vi "总圈数判定.vi"(0 "总圈数":sgl, 1 "总圈数":cluster{"下限":dbl, "上限":dbl}, 3 "错误输入":errorcluster) -> (8 "OK":bool, 10 "错误输出":errorcluster)   [LabVIEW 2018]
uses:
  Global_Variable/Global.vi
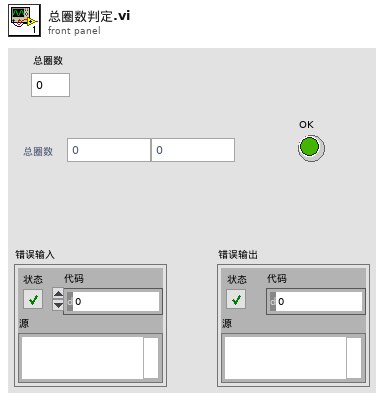
[diagram p1: front panel]
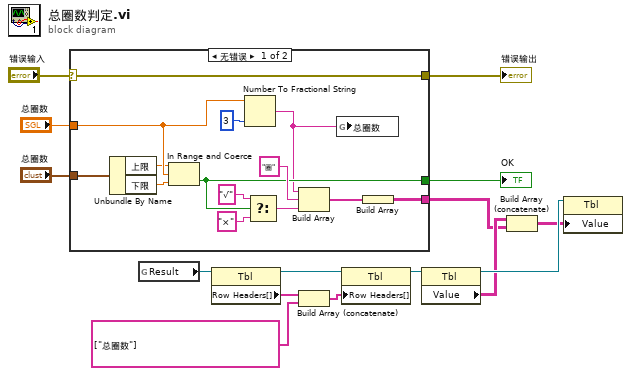
[diagram p0: block diagram]
diagram:
  n1 = case shown="无错误" "错误输入" {
    selector: "错误输入" -> [w22 w30]
    tunnel: [w22 w30] -> w14
    tunnel: [w24 _] -> w5
    tunnel: "总圈数" -> [w21 _]
    tunnel: "总圈数" -> [w20 _]
    tunnel: [w17 _] -> w1
    frame No Error {
      n2 = Unbundle By Name(w21) -> ("上限"=w19:dbl, "下限"=w18:dbl)
      n3 = In Range and Coerce(upper limit=w19, x=w20, lower limit=w18) -> (In Range?=w17:bool)  [unwired: 1 out]
      n4 = Number To Fractional String(number=w20, precision (6)=i16 3 ("精度(6)")) -> (F-format string=w16:string)  [unwired: 2 in]
      n5 = Select(t="√", s=w17, f="×") -> (s? t:f=w25:string)
      n6 = Build Array(w16, "圈" ("元素"), w25) -> (w23:string[])
      n7 = global write "检测结果.vi" "总圈数"(w16) -> ()
      n8 = Build Array(w23) -> (w24:string[][])
    }
    frame Error {
    }
  }
  "错误输出" <- w14
  "OK" <- w1
  n9 = global read "Global.vi" "Result"() -> (w13:refnum<vi>)
  n10 = property class="Tbl"(reference=w13) -> (reference out=w9:refnum<vi>, "Row Headers[]"=w12:string[])  [unwired: 1 in, 1 out]
  n11 = Build Array (concatenate)(w12, string[] ["总圈数"] ("元素")) -> (w10:string[])
  n12 = property class="Tbl"(reference=w9, "Row Headers[]"=w10) -> (reference out=w8:refnum<vi>)  [unwired: 1 in, 1 out]
  n13 = property class="Tbl"(reference=w8) -> (reference out=w7:refnum<vi>, "Value"=w6:string[][])  [unwired: 1 in, 1 out]
  n14 = Build Array (concatenate)(w6, w5) -> (w4:string[][])
  n15 = property class="Tbl"(reference=w7, "Value"=w4) -> ()  [unwired: 1 in, 2 out]
